vi "Read Functional Data (DC Monitor).vi"(8 "error in (no error)":errorcluster, 11 "VISA resource name":refnum<visa-resource-name>) -> (0 "error out":errorcluster, 1 "DC Monitor Current":dbl, 2 "DC Monitor Voltage":dbl, 3 "VISA resource name out":refnum<visa-resource-name>)   [LabVIEW 2016, in "Agilent E4980.lvlib"]
doc: "Returns the latest measured data for the DC voltage and DC current monitor. \n\n<B>Notes:</B>\n(1) If you turn OFF the voltage-level monitor, the instrument returns 0.0 to <B>DC Monitor Voltage</B>.\n\n(2) If you turn OFF the current-level monitor, the instrument returns 0.0 to <B>DC Monitor Current</B>."
uses:
  <instrlib>/Agilent E4980/Agilent E4980.lvlib
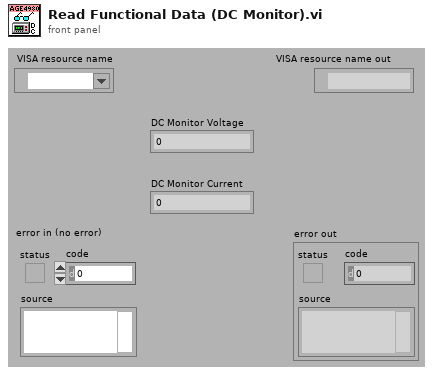
[diagram p1: front panel]
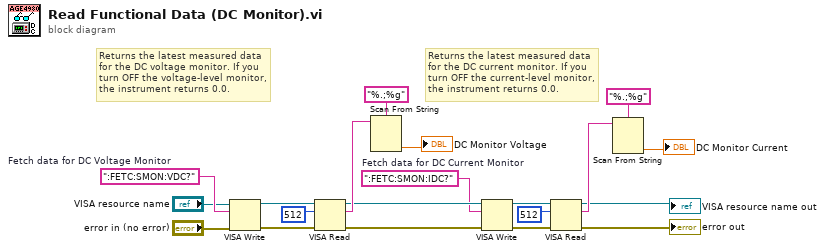
[diagram p0: block diagram]
diagram:
  w9 = ":FETC:SMON:IDC?"  # Fetch data for DC Current Monitor
  w20 = ":FETC:SMON:VDC?"  # Fetch data for DC Voltage Monitor
  # "Returns the latest measured data\nfor the DC current monitor. If you\nturn OFF the current-level monitor,\nthe instrument returns 0.0."
  # "Returns the latest measured data\nfor the DC voltage monitor. If you\nturn OFF the voltage-level monitor,\nthe instrument returns 0.0."
  n1 = VISA Write(VISA resource name="VISA resource name", write buffer=w20, error in (no error)="error in (no error)") -> (VISA resource name out=w17:refnum<visa-resource-name>, error out=w16:errorcluster)  [unwired: 1 out]
  n2 = VISA Read(VISA resource name=w17, byte count=u32 512, error in (no error)=w16) -> (VISA resource name out=w11:refnum<visa-resource-name>, read buffer=w14:string, error out=w10:errorcluster)  [unwired: 1 out]
  n3 = Scan From String(format string="%.;%g", input string=w14) -> (output 1=→"DC Monitor Voltage":dbl)  [unwired: 3 in, 3 out]
  n4 = VISA Write(VISA resource name=w11, write buffer=w9, error in (no error)=w10) -> (VISA resource name out=w8:refnum<visa-resource-name>, error out=w7:errorcluster)  [unwired: 1 out]
  n5 = VISA Read(VISA resource name=w8, byte count=u32 512, error in (no error)=w7) -> (VISA resource name out=→"VISA resource name out":refnum<visa-resource-name>, read buffer=w4:string, error out=→"error out":errorcluster)  [unwired: 1 out]
  n6 = Scan From String(format string="%.;%g", input string=w4) -> (output 1=→"DC Monitor Current":dbl)  [unwired: 3 in, 3 out]
